vi "XYZChangetoArray.vi"(3 "N pics captured":i32=10, 4 "z change":dbl, 5 "y change":dbl, 6 "x change":dbl) -> (1 "Array of Coords to go to":dbl[][](array[numeric]))   [LabVIEW 2016]
panel:
  in  "N tooling pin points":i32=8
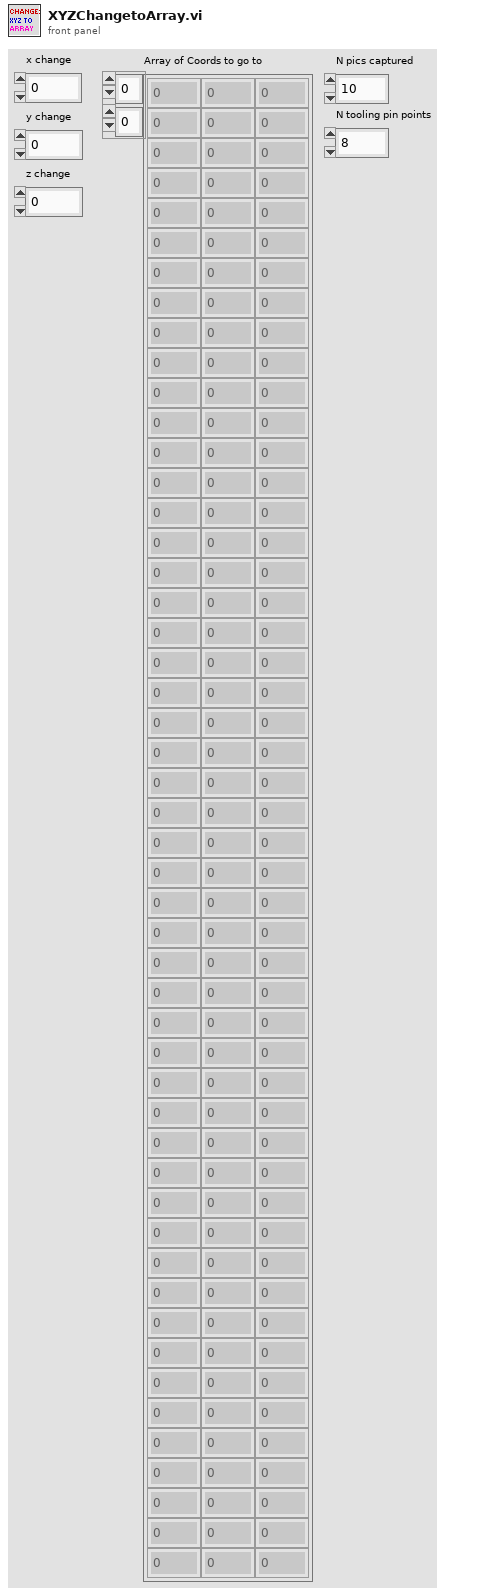
[diagram p1: front panel]
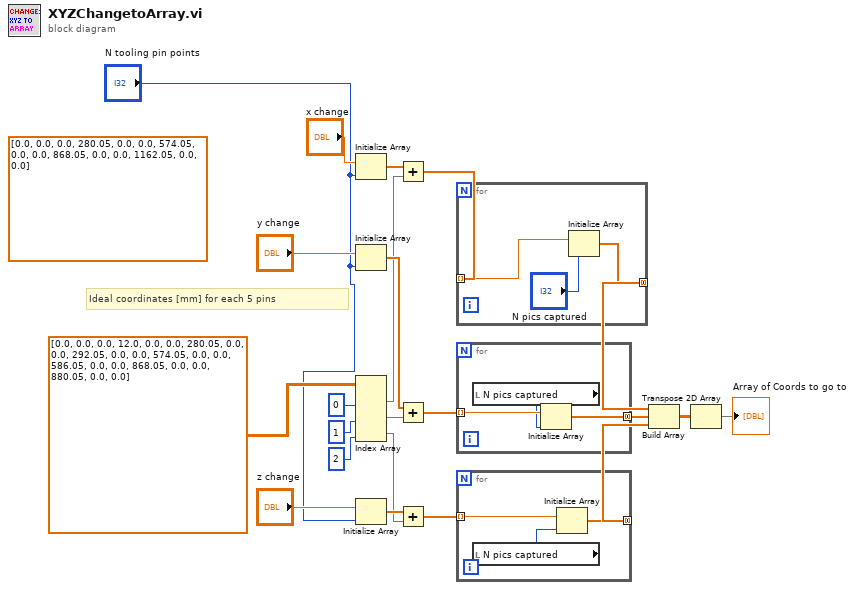
[diagram p0: block diagram]
diagram:
  (unwired) dbl[][] [[0.0, 0.0, 0.0], [280.05, 0.0, 0.0], [574.05, 0.0, 0.0], [868.05, 0.0, 0.0], [1162.05, 0.0, 0.0]] ("Set of Coordinates to Process")
  # "Ideal coordinates [mm] for each 5 pins"
  n1 = Initialize Array("x change", "N tooling pin points") -> (w17:dbl[])
  n2 = Initialize Array("y change", "N tooling pin points") -> (w16:dbl[])
  n3 = Index Array(array=dbl[][] [[0.0, 0.0, 0.0], [12.0, 0.0, 0.0], [280.05, 0.0, 0.0], [292.05, 0.0, 0.0], [574.05, 0.0, 0.0], [586.05, 0.0, 0.0], [868.05, 0.0, 0.0], [880.05, 0.0, 0.0]] ("Set of Coordinates to Process"), index (col) #1=0 ("disabled index (col)"), index (col) #2=1 ("index (col)"), index (col) #3=2 ("index (col)")) -> (element #1=w8:dbl[], element #2=w5:dbl[], element #3=w4:dbl[])  [unwired: 3 in]
  n4 = Initialize Array("z change", "N tooling pin points") -> (w15:dbl[])
  n5 = Add(x=w17, y=w8) -> (x+y=w9:dbl[])
  n6 = Add(x=w16, y=w5) -> (x+y=w11:dbl[])
  n7 = Add(x=w15, y=w4) -> (x+y=w10:dbl[])
  n8 = for {
    tunnel: w9 -> [w24] mode=indexing
    tunnel: [w23] -> w18 mode=concatenating
    n9 = Initialize Array(w24, "N pics captured") -> (w23:dbl[])
  }
  n10 = for {
    tunnel: w11 -> [w28] mode=indexing
    tunnel: [w27] -> w19 mode=concatenating
    n11 = local read "N pics captured"() -> (w26:i32)
    n12 = Initialize Array(w28, w26) -> (w27:dbl[])
  }
  n13 = for {
    tunnel: w10 -> [w31] mode=indexing
    tunnel: [w30] -> w20 mode=concatenating
    n14 = local read "N pics captured"() -> (w29:i32)
    n15 = Initialize Array(w31, w29) -> (w30:dbl[])
  }
  n16 = Build Array(w18, w19, w20) -> (w21:dbl[][])
  n17 = Transpose 2D Array(2D array=w21) -> (transposed array=→"Array of Coords to go to":dbl[][])
